vi "Control Panel Initialization Message.vi"(8 "error in (no error)":errorcluster, 10 "Resource":variant, 11 "Pump Controller in":refnum<class "Pump Controller.lvclass">) -> (0 "error out":errorcluster, 2 "Message":T1, 3 "Pump Controller out":refnum<class "Pump Controller.lvclass">)   [LabVIEW 2020, in "RxnRover.lvlib" / "Pump Controller.lvclass"]
doc: "Generate the initial message to send to the Pump Controller Control Panel."
uses:
  Pump Controller.lvclass
  <userlib>/RxnRover/DynamicReentrant/src/Type Defs/Message.ctl
  Pump Controller.lvclass/Pump Controller.ctl
  <userlib>/RxnRover/DynamicReentrant/Dynamic Reentrant.lvlib
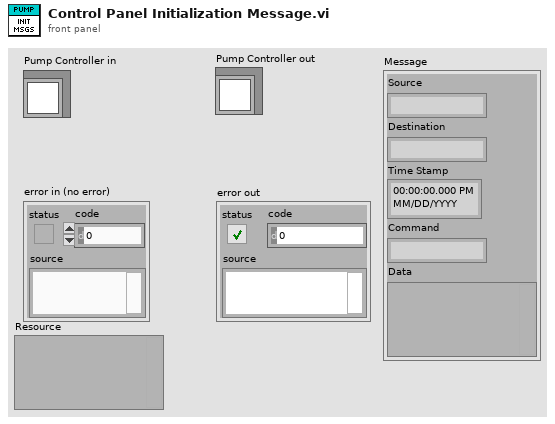
[diagram p1: front panel]
types:
  T1 = typedef "Dynamic Reentrant.lvlib/Message.ctl" = cluster{"Source":string, "Destination":string, "Time Stamp":timestamp, "Command":string, "Data":variant}
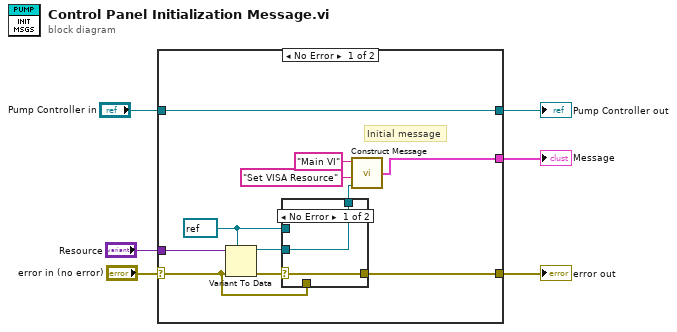
[diagram p0: block diagram]
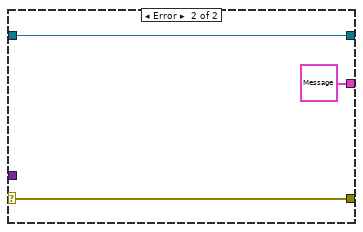
[diagram p3: hidden frame]
diagram:
  n1 = case shown="No Error" "error in (no error)" {
    selector: "error in (no error)" -> [w9 w23]
    tunnel: [w15 T1 {"Source"="", "Destination"="", "Time Stamp"=timestamp(0 s since 1904-01-01), "Command"="", "Data"=variant} ("output cluster")] -> w6
    tunnel: [w8 w23] -> w4
    tunnel: "Pump Controller in" -> [w14 w24]
    tunnel: [w14 w24] -> w2
    tunnel: "Resource" -> [w13 _]
    frame No Error {
      w11 = refnum<visa-resource-name> refnum ("VISA resource name out")
      # "Initial message"
      n2 = Variant To Data(error in=w9, type=w11, Variant=w13) -> (data=w10:refnum<visa-resource-name>, error out=w12:errorcluster)
      n3 = case shown="No Error" w12 {
        selector: w12 -> [w18 _]
        tunnel: w11 -> [_ w21]
        tunnel: w10 -> [w19 _]
        tunnel: [w19 w21] -> w7
        tunnel: [w18 w20] -> w8
        tunnel: w9 -> [_ w20]
        frame No Error {
        }
        frame Error {
        }
      }
      n4 = call <userlib>:"Construct Message.vi"("Data"=w7, "Command"="Set VISA Resource", "Source"="Main VI") -> ("Message Cluster"=w15:T1)  [unwired: 3 in]
    }
    frame Error {
    }
  }
  "Pump Controller out" <- w2
  "error out" <- w4
  "Message" <- w6
